vi "DebugLogSpeed.vi"(8 "positions [s]":dbl[](array[numeric]), 9 "t0":dbl, 11 "Instant RPM":dbl) -> ()   [LabVIEW 2017, in "CmsVirtualChannel.lvlib"]
uses:
  <vilib>/addons/InsightCM/Devices/Shared/Cms/CmsVirtualChannel/CmsVirtualChannel.lvlib
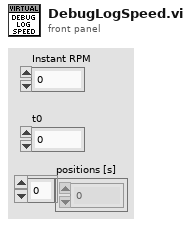
[diagram p1: front panel]
types:
  T1 = cluster{"speed":dbl, "start":dbl, "positions":dbl[]}[]
  T2 = cluster{"speed":dbl, "start":dbl, "positions":dbl[]}
  T3 = enum16{"open", "replace", "create", "open or create", "replace or create", "replace or create with confirmation"}
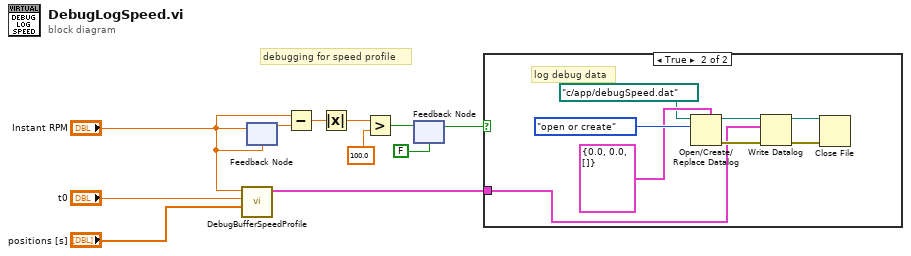
[diagram p0: block diagram]
diagram:
  # "debugging for speed profile"
  n1 = call <vilib>:"DebugBufferSpeedProfile.vi"("positions"="positions [s]", "start"="t0", "speed"="Instant RPM") -> ("speed history"=w8:T1)  [unwired: 8 in]
  n2 = feedback #1("Instant RPM") -> (w1:dbl)
  n3 = feedback-in #1("Instant RPM") -> ()
  n4 = Subtract(x="Instant RPM", y=w1) -> (x-y=w2:dbl)
  n5 = Absolute Value(x=w2) -> (abs(x)=w3:dbl)
  n6 = Greater?(x=w3, y=100.0) -> (0:w9:bool)
  n7 = feedback #2(FALSE) -> (w10:bool)
  n8 = feedback-in #2(w9) -> ()
  n9 = case shown="True" w10 {
    tunnel: w8 -> [_ w13]
    frame False {
      # "do nothing"
    }
    frame True {
      # "log debug data"
      n10 = Open/Create/Replace Datalog(5:T2 {"speed"=0.0, "start"=0.0, "positions"=[]}, 10:T3."open or create" ("operation (0:open)"), 11:path "c:/app/debugSpeed.dat" ("datalog path (use dialog)")) -> (0:w18:errorcluster, 3:w14:refnum<k1>)  [unwired: 3 in, 1 out]
      n11 = Write Datalog(4:w18, 6:w13, 7:w14) -> (0:w17:errorcluster, 3:w16:refnum<k1>)
      n12 = Close File(refnum=w16, error in=w17) -> ()  [unwired: 2 out]
    }
  }
